vi "IMAQ Dispose Buffer.vi"(2 "error in":errorcluster, 3 "Img Buffer In":T1[](array[typedef])) -> (0 "error out":errorcluster)   [LabVIEW 2013]
uses:
  <vilib>/vision/Image Controls.llb/IMAQ Image.ctl
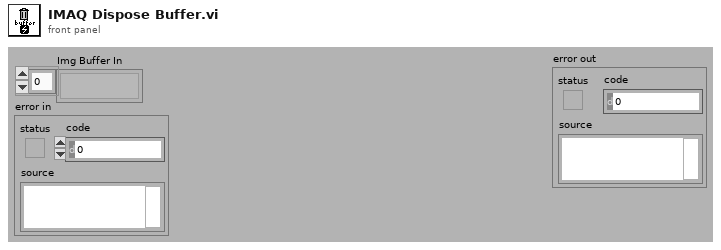
[diagram p1: front panel]
types:
  T1 = typedef "IMAQ Image.ctl" = refnum<image>
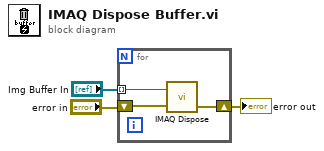
[diagram p0: block diagram]
diagram:
  n1 = for {
    tunnel: "Img Buffer In" -> [w6] mode=indexing
    shift-right: [w4] -> w1
    shift-left: "error in" -> [w5]
    n2 = call "IMAQ Dispose"("Image"=w6, "error in (no error)"=w5) -> ("error out"=w4:errorcluster)  [unwired: 1 in, 3 out]
  }
  "error out" <- w1
